vi "SVT Cross Spectrum (Real-Im).vi"(0 "scaled signal X [EUx]":waveform(dbl), 1 "scaled signal Y [EUy]":waveform(dbl), 3 "window":T10=1 items=["None"=0, "Hanning"=1, "Hamming"=2, "Blackman-Harris"=3, "Exact Blackman"=4, "Blackman"=5, "Flat Top"=6, "4 Term B-Harris "=7, "7 Term B-Harris"=8, "Low Sidelobe"=9, "Force - Exponential"=10, "Blackman Nuttall"=11, "Triangle"=30, "Bartlett-Hanning"=31, "Bohman"=32, "Parzen"=33, "Welch"=34, "Kaiser"=60, "Dolph-Chebyshev"=61, "Gaussian"=62], 5 "error in (no error)":errorcluster, 7 "averaging parameters":T9={"averaging mode"=enum."No averaging", "weighting mode"=enum."Exponential", "number of averages"=10, "linear mode"=enum."One shot"}, 8 "force/exp settings":T7={"force window [%]"=50.0, "exp window [%]"=10.0} {"exp window [%]" min=0.0 max=100.0 format="%.2f"; "force window [%]" min=0.0 max=100.0 format="%.2f"}, 9 "restart averaging (F)":bool) -> (11 "averaging done":bool, 13 "averages completed":dbl, 14 "real part [EUx EUy rms]":cluster{"f0":dbl, "df":dbl, "real part":dbl[]} {"real part" format="%.2f"; "df" format="%.2f"; "f0" format="%.2f"}, 16 "imaginary part [EUx EUy rms]":T8 {"imaginary part" format="%.2f"; "df" format="%.2f"; "f0" format="%.2f"}, 17 "unit label":string, 18 "spectrum info":T1={"channel name"="", "description"="", "x-axis units"=0, "spectral info"={"spectrum type"=enum."Power [Magnitude^2]", "linear/dB"=enum."linear", "window"=0, "window size"=0, "FFT size"=0}, "engineering units"=0, "custom label"="", "dB reference [EU]"=0.0, "peak units"=enum."rms", "weighting filter"=0, "spectral density?"=FALSE, "unit label"="", "spectrum skewed?"=FALSE, "complimentary spectrum units"=enum."none"} {"x-axis units" items=["Time (s)"=0, "Frequency-CB (Hz)"=1, "Frequency-CPB (Hz)"=1248, "Frequency-Arbitrary (Hz)"=2357, "Quefrency (s)"=2, "Revolutions (rev)"=3, "Order"=4, "Speed (RPM)"=11, "Speed (rad/s)"=21, "Index"=65535]; "weighting filter" items=["Linear", "A-weighting", "B-weighting", "C-weighting", "ITU-R 468-4", "Dolby", "CCITT", "C-message", "Wb", "Wc", "Wd", "We", "Wf", "Wh", "Wj", "Wk", "Wm", "AES17 20 kHz lowpass", "AES17 40 kHz lowpass", "AES17 20 kHz highpass", "AES17 40 kHz highpass"]; "dB reference [EU]" format="%.2f"; "engineering units" items=["custom..."=0, "V"=1, "A"=21, "C"=30, "pC"=31, "s"=32, "-"=29, "Pa"=2, "N"=20, "g"=3, "m/s^2"=4, "m/s"=5, "m"=6, "mm/s"=12, "mm"=13, "micron/s"=14, "micron"=15, "in/s^2"=7, "in/s"=8, "in"=9, "mil/s"=10, "mil"=11, "rad/s^2"=16, "rad/s"=17, "rad"=18, "deg/s^2"=26, "deg/s"=27, "deg"=28, "RPM"=22, "cycle/s^2"=23, "Hz"=24, "cycle"=25, "strain"=19]; "spectral info"."window" items=["None "=0, "Hanning"=1, "Hamming"=2, "Blackman-Harris"=3, "Exact Blackman"=4, "Blackman"=5, "Flat Top"=6, "4 Term B-Harris "=7, "7 Term B-Harris"=8, "Low Sidelobe"=9, "Force - Exponential"=10, "Gaussian"=62]}, 19 "error out":errorcluster)   [LabVIEW 2017]
doc: "Computes the cross power spectrum of <B>scaled signal X [EUx]</B> and <B>scaled signal Y [EUy]</B>. Results are returned in <B>real part [EUx EUy rms]</B> and <B>imaginary part [EUx EUy rms]</B>."
uses:
  <vilib>/addons/_NISVFA/_Shared subVIs/Controls/svc_Window [Dual FFT].ctl
  <vilib>/addons/_NISVFA/_Shared subVIs/Controls/svc_Spectrum Info.ctl
  <vilib>/addons/_NISVFA/_Shared subVIs/Controls/svc_X-Axis Units.ctl
  <vilib>/addons/_NISVFA/_Shared subVIs/Controls/svc_Spectrum Type.ctl
  <vilib>/addons/_NISVFA/_Shared subVIs/Controls/svc_Engineering Units Text Ring.ctl
  <vilib>/addons/_NISVFA/_Shared subVIs/Controls/svc_Weighting Filter Text Ring.ctl
  <vilib>/addons/_NISVFA/_Shared subVIs/Controls/svc_Complimentary Spectrum Units.ctl
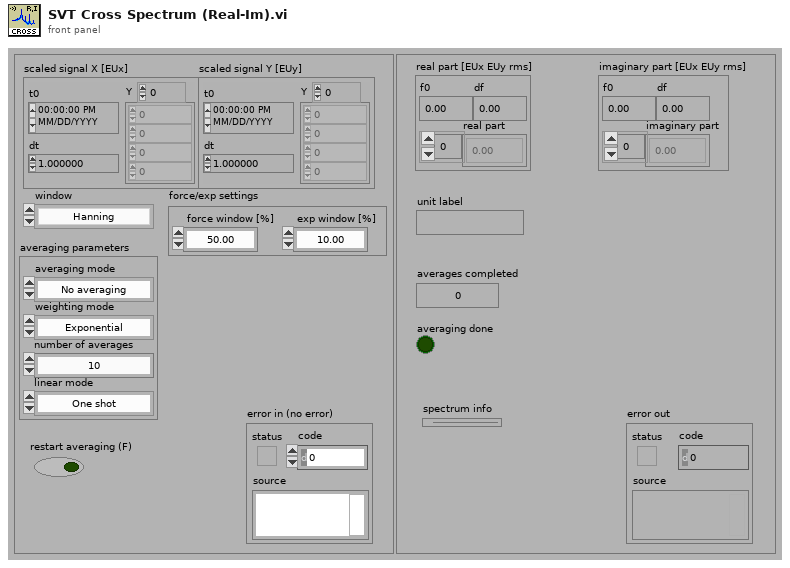
[diagram p1: front panel]
types:
  T1 = typedef "svc_Spectrum Info.ctl" = cluster{"channel name":string, "description":string, "x-axis units":T2, "spectral info":cluster{"spectrum type":T3, "linear/dB":enum16{"linear", "dB"}, "window":u16, "window size":i32, "FFT size":i32}, "engineering units":T4, "custom label":string, "dB reference [EU]":dbl, "peak units":enum16{"rms", "peak", "peak-peak"}, "weighting filter":T5, "spectral density?":bool, "unit label":string, "spectrum skewed?":bool, "complimentary spectrum units":T6}
  T2 = typedef "svc_X-Axis Units.ctl" = u16
  T3 = typedef "svc_Spectrum Type.ctl" = enum16{"FFT Spectrum [complex]", "Amplitude [Magnitude]", "Power [Magnitude^2]", "Cross Spectrum [complex]", "Frequency Response [Complex]"}
  T4 = typedef "svc_Engineering Units Text Ring.ctl" = u16
  T5 = typedef "svc_Weighting Filter Text Ring.ctl" = u16
  T6 = typedef "svc_Complimentary Spectrum Units.ctl" = enum16{"none", "radians", "degrees", "cycles", "imaginary"}
  T7 = cluster{"force window [%]":dbl, "exp window [%]":dbl}
  T8 = cluster{"f0":dbl, "df":dbl, "imaginary part":dbl[]}
  T9 = cluster{"averaging mode":enum16{"No averaging", "Vector averaging", "RMS averaging", "Peak hold"}, "weighting mode":enum16{"Linear", "Exponential"}, "number of averages":u32, "linear mode":enum16{"One shot", "Auto restart"}}
  T10 = typedef "svc_Window [Dual FFT].ctl" = u32
  T11 = enum16{"Cross spectrum", "Frequency response", "Coherent output power"}
  T12 = enum16{"Restart processing", "Continue processing", "Skip processing"}
  T13 = cluster{"f0":dbl, "df":dbl, "complex spectrum":cdb[]}
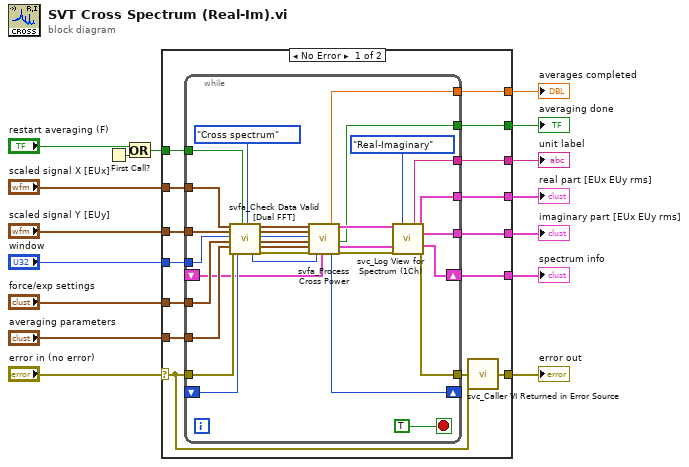
[diagram p0: block diagram]
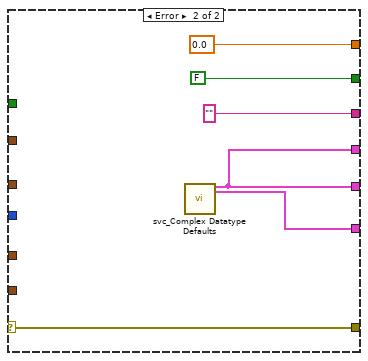
[diagram p2: hidden frame]
diagram:
  n1 = First Call?() -> (First Call?: T/F=w3:bool)
  n2 = Or(x="restart averaging (F)", y=w3) -> (x .or. y?=w1:bool)
  n3 = case shown="No Error" "error in (no error)" {
    selector: "error in (no error)" -> [w17 w67]
    tunnel: "window" -> [w29 _]
    tunnel: "averaging parameters" -> [w27 _]
    tunnel: [w18 w67] -> w14
    tunnel: [w25 w62] -> w13
    tunnel: "force/exp settings" -> [w28 _]
    tunnel: "scaled signal X [EUx]" -> [w26 _]
    tunnel: "scaled signal Y [EUy]" -> [w30 _]
    tunnel: w1 -> [w21 _]
    tunnel: [w31 "" ("Unit label [Mag - Real]")] -> w8
    tunnel: [w22 0.0 ("averages completed")] -> w7
    tunnel: [w23 FALSE ("averaging done")] -> w6
    tunnel: [w24 w62] -> w5
    tunnel: [w19 w63] -> w4
    frame No Error {
      n4 = while {
        tunnel: [w38] -> w20
        tunnel: w21 -> [w39]
        shift-left: _ -> [w41]
        shift-right: [w40] -> _
        tunnel: [w42] -> w22
        tunnel: [w43] -> w23
        tunnel: [w44] -> w24
        tunnel: [w45] -> w25
        tunnel: w26 -> [w47]
        tunnel: w17 -> [w48]
        tunnel: w27 -> [w49]
        tunnel: w28 -> [w50]
        tunnel: w29 -> [w51]
        tunnel: w30 -> [w52]
        tunnel: [w53] -> w31
        shift-right: [w37] -> w19
        shift-left: _ -> [w32]
        stop <- TRUE stop-if-true
        n5 = call <vilib>:"svfa_Check Data Valid [Dual FFT].vi"("stimulus [X]"=w47, "response [Y]"=w52, "window"=w51, "force/exp settings"=w50, "averaging parameters"=w49, "error in (no error)"=w48, "processing control in"=w41, "restart averaging (F)"=w39, "measurement"=T11."Cross spectrum") -> ("processing control out"=w35:T12, "dup stimulus [X]"=w61:waveform(dbl), "dup response [Y]"=w59:waveform(dbl), "window"=w58:T10, "dup force/exp settings"=w57:T7, "dup averaging parameters"=w56:T9, "error out"=w55:errorcluster)  [unwired: 3 in, 1 out]
        n6 = call <vilib>:"svfa_Process Cross Power.vi"("input signal X"=w61, "input signal Y"=w59, "window"=w58, "force/exp settings"=w57, "averaging parameters"=w56, "error in (no error)"=w55, "processing control in"=w35, "spectrum info in"=w32) -> ("averages completed"=w42:dbl, "processing control out"=w40:T12, "complex spectrum"=w60:T13, "averaging done"=w43:bool, "spectrum info out"=w33:T1, "error out"=w34:errorcluster)  [unwired: 6 in]
        n7 = call <vilib>:"svc_Log View for Spectrum (1Ch).vi"("complex spectrum"=w60, "View"=enum16{"Mag-Phase", "Real-Imaginary"}."Real-Imaginary", "spectrum info in"=w33, "error in (no error)"=w34) -> ("unit label [mag or real]"=w53:string, "magnitude or real"=w44:cluster{"f0":dbl, "df":dbl, dbl[]}, "phase or imag"=w45:cluster{"f0":dbl, "df":dbl, dbl[]}, "spectrum info out"=w37:T1, "error out"=w38:errorcluster)  [unwired: 6 in, 1 out]
      }
      n8 = call <vilib>:"svc_Caller VI Returned in Error Source.vi"("warning input to caller"=w17, "error in (no error)"=w20) -> ("error out"=w18:errorcluster)  [unwired: 3 in]
    }
    frame Error {
      n9 = call <vilib>:"svc_Complex Datatype Defaults.vi"() -> ("empty spectrum"=w62:cluster{"f0":dbl, "df":dbl, "magnitude":dbl[]}, "dead spectrum info"=w63:T1)  [unwired: 11 in, 7 out]
    }
  }
  "error out" <- w14
  "imaginary part [EUx EUy rms]" <- w13
  "real part [EUx EUy rms]" <- w5
  "unit label" <- w8
  "averages completed" <- w7
  "averaging done" <- w6
  "spectrum info" <- w4
